vi "get_or_set_dimension.vi"(5 "dimension":T2, 6 "number of pixels to get (-1: get all)":i32=-1, 7 "action":T1, 8 "error in (no error)":errorcluster, 10 "pixel values in (single dimension)":dbl[unit][](array[numeric]), 11 "GenericTrajectory in":refnum<class "TrajectoryDL091126GenericVoxel.lvclass">) -> (0 "error out":errorcluster, 2 "pixel values out (single dimension)":dbl[unit][](array[numeric]), 3 "GenericTrajectory out":refnum<class "TrajectoryDL091126GenericVoxel.lvclass">)   [LabVIEW 2010, in "TrajectoryDL091126GenericVoxel.lvclass"]
uses:
  TrajectoryDL091126GenericVoxel.lvclass
  common/enumerations/x_y_z_enumeration.ctl
  common/enumerations/functional_global_action_enum.ctl
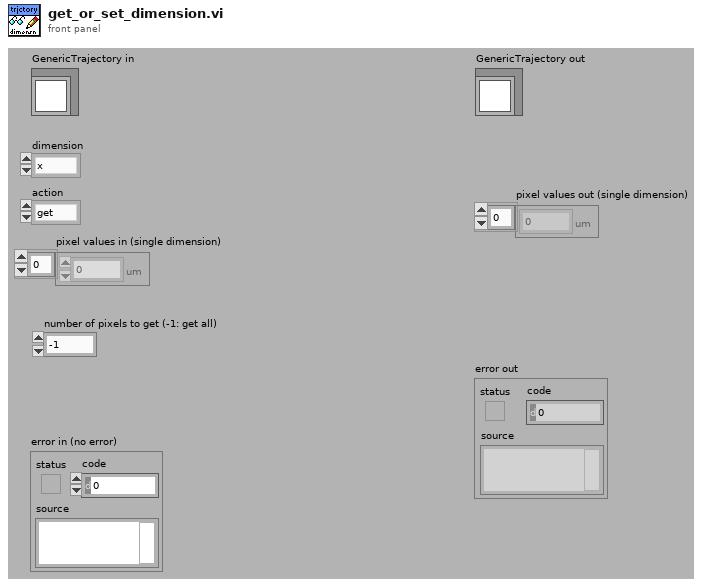
[diagram p1: front panel]
types:
  T1 = typedef "functional_global_action_enum.ctl" = enum16{"get", "set", "reset"}
  T2 = typedef "x_y_z_enumeration.ctl" = enum16{"x", "y", "z"}
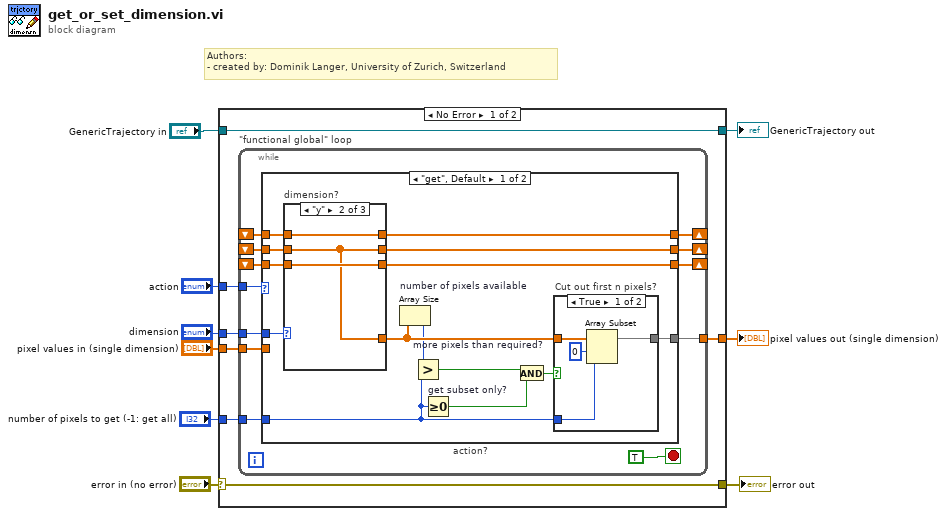
[diagram p0: block diagram]
diagram:
  # "Authors: \n- created by: Dominik Langer, University of Zurich, Switzerland"
  n1 = case shown="No Error" "error in (no error)" {
    selector: "error in (no error)" -> [w16 w75]
    tunnel: [w16 w75] -> w8
    tunnel: [w14 w74] -> w6
    tunnel: "GenericTrajectory in" -> [w14 w74]
    tunnel: "dimension" -> [w15 _]
    tunnel: [w13 _] -> w2
    tunnel: "action" -> [w12 _]
    tunnel: "pixel values in (single dimension)" -> [w11 _]
    tunnel: "number of pixels to get (-1: get all)" -> [w10 _]
    frame No Error {
      n2 = while "\"functional global\" loop" {
        tunnel: w15 -> [w28]
        tunnel: [w27] -> w13
        tunnel: w12 -> [w20]
        shift-right: [w23] -> _
        shift-left: _ -> [w26]
        shift-right: [w22] -> _
        shift-left: _ -> [w25]
        shift-right: [w21] -> _
        shift-left: _ -> [w24]
        tunnel: w11 -> [w19]
        tunnel: w10 -> [w17]
        stop <- TRUE stop-if-true
        n3 = case "action?" shown="\"get\", Default" w20 {
          tunnel: w28 -> [w42 w64]
          tunnel: [w35 _] -> w27
          tunnel: w26 -> [w41 w63]
          tunnel: w25 -> [w38 w62]
          tunnel: w24 -> [w39 w61]
          tunnel: [w40 w60] -> w23
          tunnel: [w37 w59] -> w22
          tunnel: [w36 w58] -> w21
          tunnel: w19 -> [_ w57]
          tunnel: w17 -> [w29 _]
          frame "get", Default {
            n4 = case "dimension?" shown="\"y\"" w42 {
              tunnel: [w48 w51 w54] -> w34
              tunnel: w41 -> [w48 w53 w56]
              tunnel: [w48 w53 w56] -> w40
              tunnel: w39 -> [w49 w52 w54]
              tunnel: w38 -> [w50 w51 w55]
              tunnel: [w50 w51 w55] -> w37
              tunnel: [w49 w52 w54] -> w36
              frame "x", Default {
              }
              frame "y" {
              }
              frame "z" {
              }
            }
            n5 = Array Size "number of pixels available"(array=w34) -> (size(s)=w33:i32)
            n6 = Greater? "more pixels than required?"(x=w33, y=w29) -> (0:w31:bool)
            n7 = Greater Or Equal To 0? "get subset only?"(x=w29) -> (x >= 0?=w32:bool)
            n8 = And(x=w31, y=w32) -> (x .and. y?=w30:bool)
            n9 = case "Cut out first n pixels?" shown="True" w30 {
              tunnel: w34 -> [w44 w47]
              tunnel: [w46 w47] -> w35
              tunnel: w29 -> [w43 _]
              frame True {
                n10 = Array Subset(array=w44, index=0, length=w43) -> (w46:dbl[unit][])
              }
              frame False {
              }
            }
          }
          frame "set" {
            n11 = case "dimension?" shown="\"z\"" w64 {
              tunnel: w63 -> [_ w68 w71]
              tunnel: w62 -> [w67 _ w72]
              tunnel: w61 -> [w66 w69 _]
              tunnel: [w65 w68 w71] -> w60
              tunnel: [w67 w70 w72] -> w59
              tunnel: [w66 w69 w73] -> w58
              tunnel: w57 -> [w65 w70 w73]
              frame "x", Default {
              }
              frame "y" {
              }
              frame "z" {
              }
            }
          }
        }
      }
    }
    frame Error {
    }
  }
  "error out" <- w8
  "GenericTrajectory out" <- w6
  "pixel values out (single dimension)" <- w2
